vi "escribe_tbl_instrumento.vi"(8 "error in (no error)":errorcluster, 10 "cluster_equipos":T1, 11 "DB in":refnum<class "Base de Datos.lvclass">) -> (0 "error out":errorcluster, 3 "object out":refnum<class "Base de Datos.lvclass">)   [LabVIEW 2019, in "Base de Datos.lvclass"]
uses:
  Base de Datos.lvclass
  SQLiteConnector/SQLiteConnection.lvclass
  Controles/cluster_equipos.ctl
panel:
  out "Paso 1":string
  # "Tabla que registra los datos del equipo a ingresar"
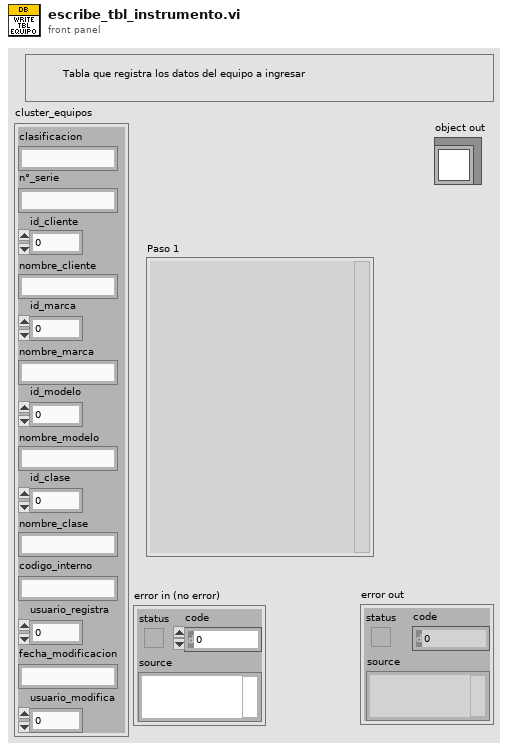
[diagram p1: front panel]
types:
  T1 = typedef "Base de Datos.lvclass/cluster_equipos.ctl" = cluster{"clasificacion":string, "n°_serie":string, "id_cliente":i32, "nombre_cliente":string, "id_marca":i32, "nombre_marca":string, "id_modelo":i32, "nombre_modelo":string, "id_clase":i32, "nombre_clase":string, "codigo_interno":string, "usuario_registra":i32, "fecha_modificacion":string, "usuario_modifica":i32}
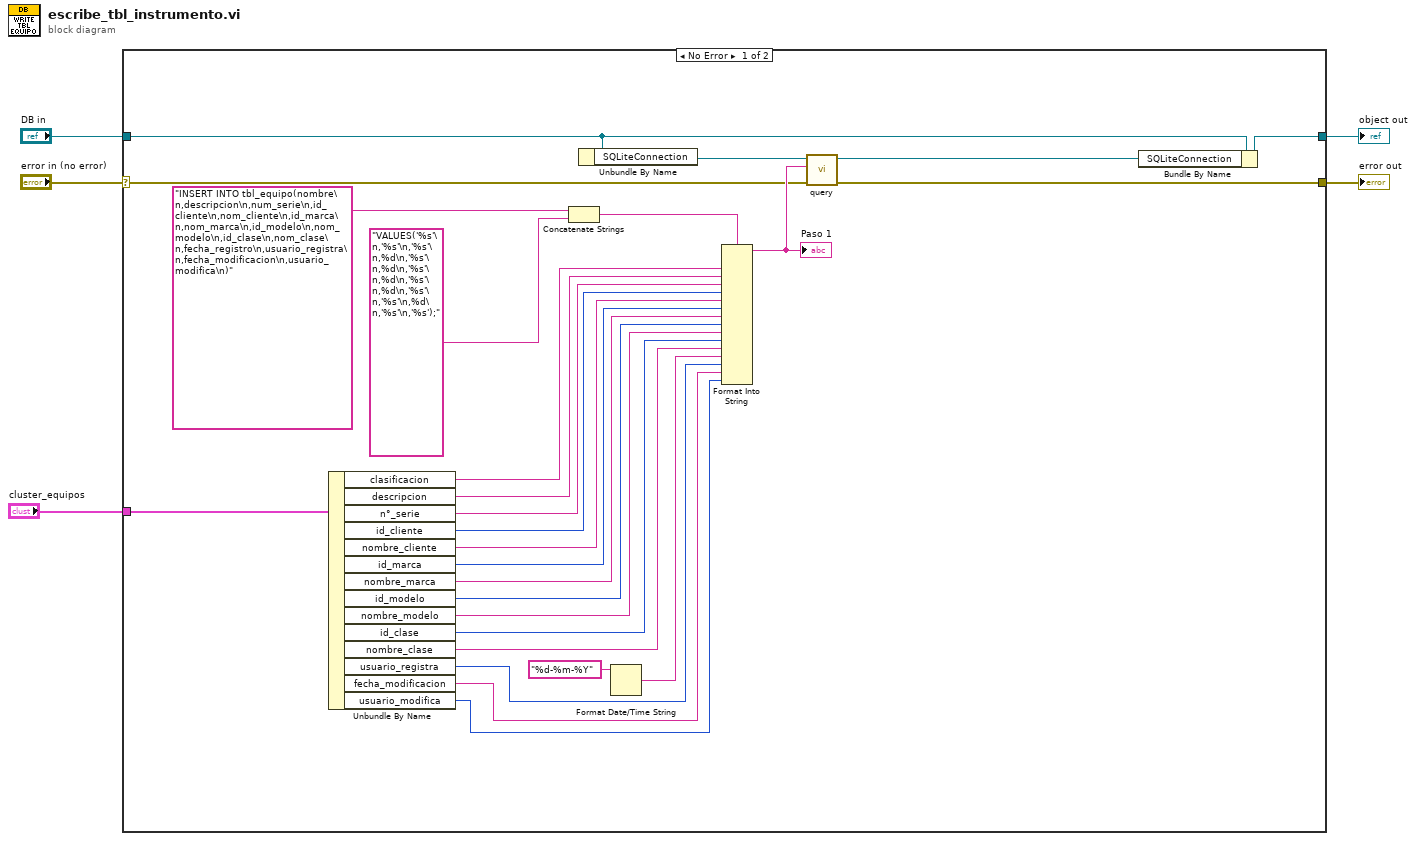
[diagram p0: block diagram]
diagram:
  n1 = case shown="No Error" "error in (no error)" {
    selector: "error in (no error)" -> [w28 w34]
    tunnel: [w29 w34] -> w5
    tunnel: "DB in" -> [w26 w33]
    tunnel: [w24 w33] -> w2
    tunnel: "cluster_equipos" -> [w21 _]
    frame No Error {
      n2 = Unbundle By Name(w21) -> ("clasificacion"=w20:string, "descripcion"=w19:string, "n°_serie"=w18:string, "id_cliente"=w17:i32, "nombre_cliente"=w16:string, "id_marca"=w15:i32, "nombre_marca"=w14:string, "id_modelo"=w13:i32, "nombre_modelo"=w12:string, "id_clase"=w11:i32, "nombre_clase"=w10:string, "usuario_registra"=w8:i32, "fecha_modificacion"=w7:string, "usuario_modifica"=w6:i32)
      n3 = Concatenate Strings("INSERT INTO tbl_equipo(nombre\n,descripcion\n,num_serie\n,id_cliente\n,nom_cliente\n,id_marca\n,nom_marca\n,id_modelo\n,nom_modelo\n,id_clase\n,nom_clase\n,fecha_registro\n,usuario_registra\n,fecha_modificacion\n,usuario_modifica\n)" ("format string"), "VALUES('%s'\n,'%s'\n,'%s'\n,%d\n,'%s'\n,%d\n,'%s'\n,%d\n,'%s'\n,%d\n,'%s'\n,'%s'\n,%d\n,'%s'\n,'%s');" ("format string")) -> (w22:string)
      n4 = Unbundle By Name(w26) -> ("SQLiteConnection"=w25:refnum<class "SQLiteConnection.lvclass">)
      n5 = Format Date/Time String(time format string (%c)="%d-%m-%Y") -> (date/time string=w9:string)  [unwired: 2 in]
      n6 = Format Into String(format string=w22, w20, w19, w18, w17, w16, w15, w14, w13, w12, w11, w10, w9, w8, w7, w6) -> (resulting string=w32:string)  [unwired: 2 in, 1 out]
      "Paso 1" <- w32
      n7 = call "query.vi"("error in (no error)"=w28, "SQL Statement"=w32, "object in"=w25) -> ("error out"=w29:errorcluster, "object out"=w27:refnum<class "SQLiteConnection.lvclass">)  [unwired: 5 in, 2 out]
      n8 = Bundle By Name(cluster=w26, "SQLiteConnection"=w27) -> (w24:refnum<class "Base de Datos.lvclass">)
    }
    frame Error {
    }
  }
  "error out" <- w5
  "object out" <- w2
